vi "Test3.vi"() -> ()   [LabVIEW 2010]
uses:
  <vilib>/MDSplus/Classes/Data_Class/Scalar_Class/Float32_Class/Float32.lvclass
  <vilib>/MDSplus/Classes/Data_Class/Data.lvclass
  <vilib>/MDSplus/Classes/Tree_Class/Tree.lvclass
  <vilib>/MDSplus/Classes/Data_Class/TreeNode_Class/TreeNode.lvclass
panel:
  out "error out":errorcluster
  in  "Value":sgl=6.6666
  in  "Path":string=":NUMX"
  in  "Mode":string="EDIT"
  in  "Shot":i32=-1
  in  "Name":string="my_tree"
  out "Float out":sgl
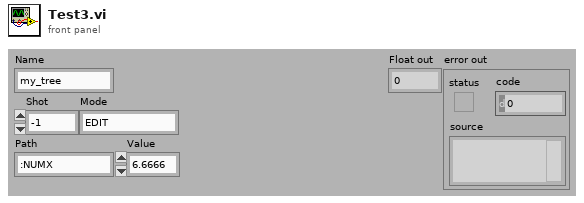
[diagram p1: front panel]
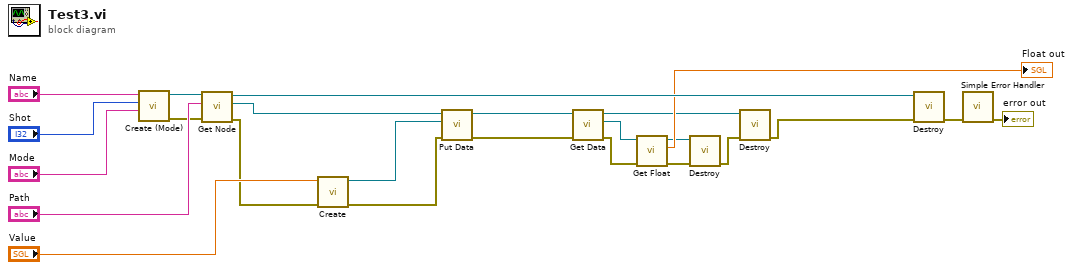
[diagram p0: block diagram]
diagram:
  n1 = call <vilib>:"Create (Mode).vi"("Mode"="Mode", "Shot"="Shot", "Name"="Name") -> ("error out"=w17:errorcluster, "Tree out"=w18:refnum<class "Tree.lvclass">)  [unwired: 7 in]
  n2 = call-dynamic "Get Node.vi"("error in (no error)"=w17, "Path"="Path", "Tree in"=w18) -> ("error out"=w11:errorcluster, "Node out"=w16:refnum<class "TreeNode.lvclass">, "Tree out"=w20:refnum<class "Tree.lvclass">)  [unwired: 6 in]
  n3 = call <vilib>:"Create.vi"("error in (no error)"=w11, "SGL in"="Value") -> ("error out"=w10:errorcluster, "Float32 out"=w2:refnum<class "Float32.lvclass">)  [unwired: 8 in]
  n4 = call-dynamic "Put Data.vi"("error in (no error)"=w10, "Data in"=w2, "TreeNode in"=w16) -> ("error out"=w1:errorcluster, "TreeNode out"=w14:refnum<class "TreeNode.lvclass">)  [unwired: 7 in]
  n5 = call-dynamic "Get Data.vi"("error in (no error)"=w1, "TreeNode in"=w14) -> ("error out"=w12:errorcluster, "Data out"=w13:refnum<class "Data.lvclass">, "TreeNode out"=w6:refnum<class "TreeNode.lvclass">)  [unwired: 7 in]
  n6 = call-dynamic "Get Float.vi"("error in (no error)"=w12, "Data in"=w13) -> ("error out"=w7:errorcluster, "SGL out"=→"Float out":sgl, "Data out"=w8:refnum<class "Data.lvclass">)  [unwired: 7 in]
  n7 = call-dynamic "Destroy.vi"("error in (no error)"=w7, "Data in"=w8) -> ("error out"=w5:errorcluster)  [unwired: 9 in]
  n8 = call-dynamic "Destroy.vi"("error in (no error)"=w5, "TreeNode in"=w6) -> ("error out"=w3:errorcluster)  [unwired: 9 in]
  n9 = call-dynamic "Destroy.vi"("error in (no error)"=w3, "Tree in"=w20) -> ("error out"=w19:errorcluster)  [unwired: 8 in]
  n10 = call <vilib>:"Simple Error Handler.vi"("error in (no error)"=w19) -> ("error out"=→"error out":errorcluster)  [unwired: 4 in, 4 out]
